vi "rot1.vi"(1 "t0":timestamp format="%<%.7X\n%x>T", 2 "input":timestamp[](array[timestamp])) -> (0 "output array":timestamp[](array[timestamp]) caption="История" format="%<%.7X>T")   [LabVIEW 2010]
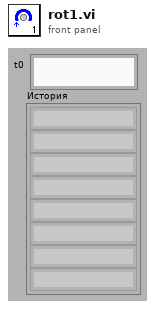
[diagram p1: front panel]
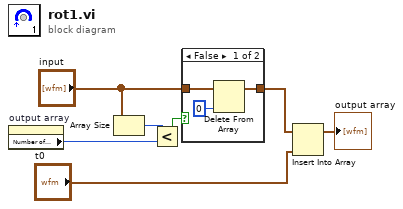
[diagram p0: block diagram]
diagram:
  n1 = property on="output array" class="Arr (strict)"() -> ("Number of Rows"=w3:u32)  [unwired: 2 in, 2 out]
  n2 = Array Size(array="input") -> (size(s)=w7:i32)
  n3 = Less?(x=w7, y=w3) -> (x < y?=w6:bool)
  n4 = case shown="False" w6 {
    tunnel: [w9 w11] -> w5
    tunnel: "input" -> [w10 w11]
    frame False {
      n5 = Delete From Array(array=w10, index=0) -> (array with subset deleted=w9:timestamp[])  [unwired: 1 in, 1 out]
    }
    frame True {
    }
  }
  n6 = Insert Into Array(array=w5, new element="t0") -> (→"output array":timestamp[])  [unwired: 1 in]
